vi "BriguyMecanumCode.vi"(0 "ErrorInBR":errorcluster, 1 "ErrorInBL":errorcluster, 2 "ErrorInFR":errorcluster, 3 "ErrorInFL":errorcluster, 4 "Rotation":dbl, 5 "Y":dbl, 7 "X":dbl, 8 "BackRight":T1={"DeviceStatus"={"status"=FALSE, "code"=0, "source"=""}, "Type"=enum."PWM", "PWM"={"Digital Module"=enum."Digital Module 1", "PWM Channel"=enum."Invalid", "DeadBand"={"Name"="", "maxPositivePwm"=0, "minPositivePwm"=0, "centerPwm"=0, "maxNegativePwm"=0, "minNegativePwm"=0, "angularRange"=0}}, "CAN"={"Device Number"=0, "Control Mode"=enum."Percent VBus", "Semaphore"=refnum, "Max Vout"=12.0}, "Invert"=FALSE, "TransformRef"=refnum, "InvTransformRef"=refnum}, 9 "BackLeft":T1={"DeviceStatus"={"status"=FALSE, "code"=0, "source"=""}, "Type"=enum."PWM", "PWM"={"Digital Module"=enum."Digital Module 1", "PWM Channel"=enum."Invalid", "DeadBand"={"Name"="", "maxPositivePwm"=0, "minPositivePwm"=0, "centerPwm"=0, "maxNegativePwm"=0, "minNegativePwm"=0, "angularRange"=0}}, "CAN"={"Device Number"=0, "Control Mode"=enum."Percent VBus", "Semaphore"=refnum, "Max Vout"=12.0}, "Invert"=FALSE, "TransformRef"=refnum, "InvTransformRef"=refnum}, 10 "FrontRight":T1={"DeviceStatus"={"status"=FALSE, "code"=0, "source"=""}, "Type"=enum."PWM", "PWM"={"Digital Module"=enum."Digital Module 1", "PWM Channel"=enum."Invalid", "DeadBand"={"Name"="", "maxPositivePwm"=0, "minPositivePwm"=0, "centerPwm"=0, "maxNegativePwm"=0, "minNegativePwm"=0, "angularRange"=0}}, "CAN"={"Device Number"=0, "Control Mode"=enum."Percent VBus", "Semaphore"=refnum, "Max Vout"=12.0}, "Invert"=FALSE, "TransformRef"=refnum, "InvTransformRef"=refnum}, 11 "FrontLeft":T1={"DeviceStatus"={"status"=FALSE, "code"=0, "source"=""}, "Type"=enum."PWM", "PWM"={"Digital Module"=enum."Digital Module 1", "PWM Channel"=enum."Invalid", "DeadBand"={"Name"="", "maxPositivePwm"=0, "minPositivePwm"=0, "centerPwm"=0, "maxNegativePwm"=0, "minNegativePwm"=0, "angularRange"=0}}, "CAN"={"Device Number"=0, "Control Mode"=enum."Percent VBus", "Semaphore"=refnum, "Max Vout"=12.0}, "Invert"=FALSE, "TransformRef"=refnum, "InvTransformRef"=refnum}) -> (6 "error out":errorcluster)   [LabVIEW 2011]
uses:
  <vilib>/Rock Robotics/WPI/MotorControl/WPI_MotorControlDeviceRef.ctl
  <vilib>/Rock Robotics/SystemInterfaces/Typedef/FPGA_TypedefDigitalModule.ctl
  <vilib>/Rock Robotics/SystemInterfaces/DIO/FPGA_DIOPWMChannel.ctl
  <vilib>/Rock Robotics/WPI/PWM/WPI_PWMDeadband.ctl
  <vilib>/Rock Robotics/WPI/CAN/Jaguar/SubVIs/WPI_CANJaguar_ControlMode.ctl
  <vilib>/Rock Robotics/WPI/PWM/WPI_PWMTransform_ConPane.ctl
panel:
  in  "Run Code?":bool=TRUE
  in  "Max Output":dbl
  in  "Gyro Angle":dbl
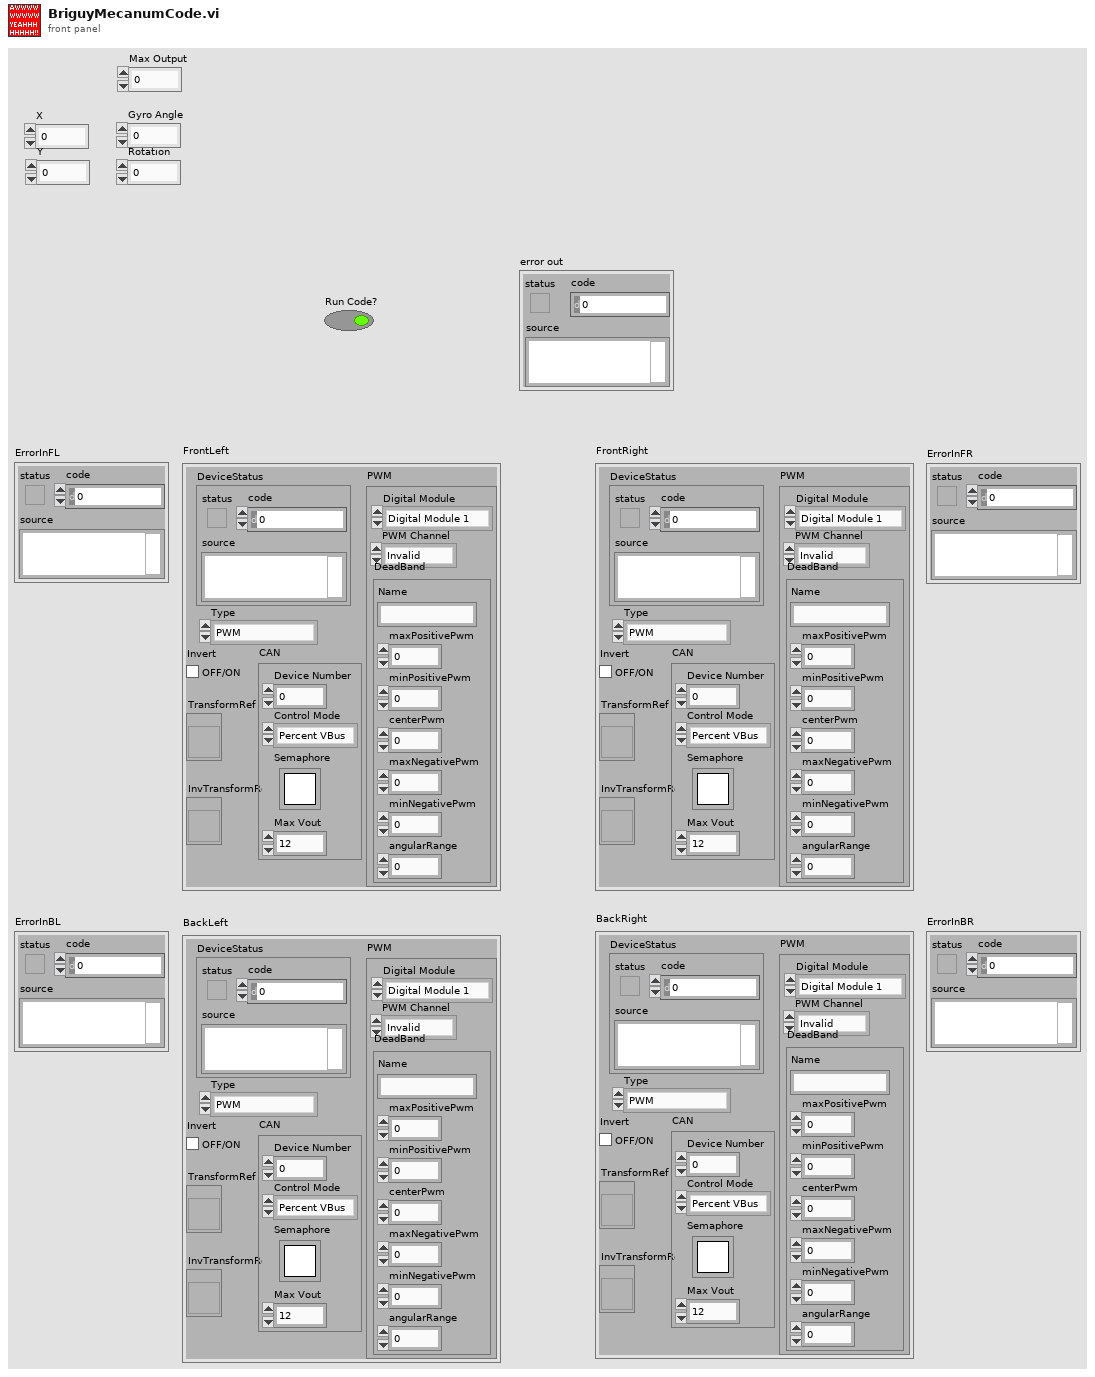
[diagram p1: front panel]
types:
  T1 = typedef "WPI_MotorControlDeviceRef.ctl" = cluster{"DeviceStatus":errorcluster, "Type":enum16{"PWM", "CAN"}, "PWM":cluster{"Digital Module":T2, "PWM Channel":T3, "DeadBand":T4}, "CAN":cluster{"Device Number":u8, "Control Mode":T5, "Semaphore":T6, "Max Vout":dbl}, "Invert":bool, "TransformRef":T7, "InvTransformRef":T7}
  T2 = typedef "FPGA_TypedefDigitalModule.ctl" = enum16{"Digital Module 1", "Digital Module 2"}
  T3 = typedef "FPGA_DIOPWMChannel.ctl" = enum8{"PWM 1", "PWM 2", "PWM 3", "PWM 4", "PWM 5", "PWM 6", "PWM 7", "PWM 8", "PWM 9", "PWM 10", "Invalid"}
  T4 = typedef "WPI_PWMDeadband.ctl" = cluster{"Name":string, "maxPositivePwm":i32, "minPositivePwm":i32, "centerPwm":i32, "maxNegativePwm":i32, "minNegativePwm":i32, "angularRange":u16}
  T5 = typedef "WPI_CANJaguar_ControlMode.ctl" = enum8{"Percent VBus", "Current", "Speed", "Position", "Voltage"}
  T6 = typedef "Semaphore RefNum" = refnum<k1>
  T7 = typedef "WPI_PWMTransform_ConPane.ctl" = refnum<vi>
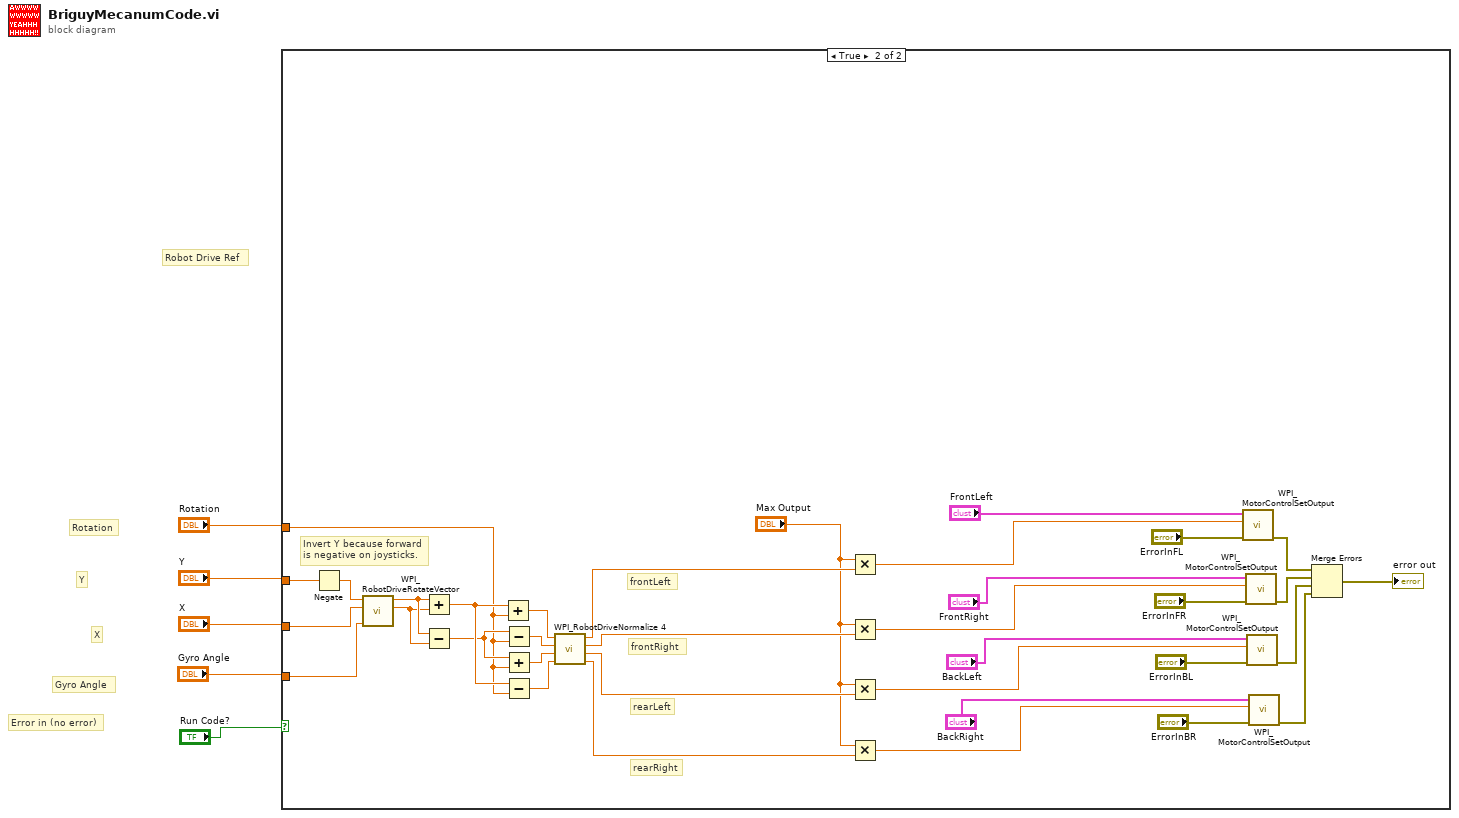
[diagram p0: block diagram]
diagram:
  # "Error in (no error)"
  # "Robot Drive Ref"
  # "Gyro Angle"
  # "X"
  # "Y"
  # "Rotation"
  n1 = case shown="True" "Run Code?" {
    tunnel: "Y" -> [_ w26]
    tunnel: "X" -> [_ w31]
    tunnel: "Rotation" -> [_ w32]
    tunnel: "Gyro Angle" -> [_ w25]
    frame False {
    }
    frame True {
      # "Invert Y because forward is negative on joysticks."
      # "rearLeft"
      # "frontRight"
      # "rearRight"
      # "frontLeft"
      n2 = Negate(x=w26) -> (-x=w24:dbl)
      n3 = call <vilib>:"WPI_RobotDriveRotateVector.vi"("Angle"=w25, "X"=w31, "Y"=w24) -> ("X'"=w39:dbl, "Y'"=w40:dbl)  [unwired: 7 out]
      n4 = Add(x=w40, y=w39) -> (x+y=w37:dbl)
      n5 = Subtract(x=w40, y=w39) -> (x-y=w35:dbl)
      n6 = Add(x=w37, y=w32) -> (x+y=w33:dbl)
      n7 = Subtract(x=w35, y=w32) -> (x-y=w34:dbl)
      n8 = Add(x=w35, y=w32) -> (x+y=w36:dbl)
      n9 = Subtract(x=w37, y=w32) -> (x-y=w38:dbl)
      n10 = call <vilib>:"WPI_RobotDriveNormalize 4.vi"("D"=w38, "C"=w36, "B"=w34, "A"=w33) -> ("D'"=w28:dbl, "C'"=w27:dbl, "B'"=w29:dbl, "A'"=w30:dbl)
      n11 = Multiply(x="Max Output", y=w30) -> (x*y=w23:dbl)
      n12 = Multiply(x="Max Output", y=w29) -> (x*y=w22:dbl)
      n13 = Multiply(x="Max Output", y=w27) -> (x*y=w21:dbl)
      n14 = Multiply(x="Max Output", y=w28) -> (x*y=w20:dbl)
      n15 = call <vilib>:"WPI_MotorControlSetOutput.vi"("error in (no error)"="ErrorInFL", "Output"=w23, "MotorControlDevRef"="FrontLeft") -> ("error out"=w11:errorcluster)  [unwired: 2 in, 6 out]
      n16 = call <vilib>:"WPI_MotorControlSetOutput.vi"("error in (no error)"="ErrorInFR", "Output"=w22, "MotorControlDevRef"="FrontRight") -> ("error out"=w17:errorcluster)  [unwired: 2 in, 6 out]
      n17 = call <vilib>:"WPI_MotorControlSetOutput.vi"("error in (no error)"="ErrorInBL", "Output"=w21, "MotorControlDevRef"="BackLeft") -> ("error out"=w18:errorcluster)  [unwired: 2 in, 6 out]
      n18 = call <vilib>:"WPI_MotorControlSetOutput.vi"("error in (no error)"="ErrorInBR", "Output"=w20, "MotorControlDevRef"="BackRight") -> ("error out"=w19:errorcluster)  [unwired: 2 in, 6 out]
      n19 = Merge Errors(w11, w17, w18, w19) -> (→"error out":errorcluster)
    }
  }
